vi "PickAndDestroy.vi"(0 "Image Settings":T3 {"2nd Axis" items=["x", "y", "z"]; "1st Axis" items=["x", "y", "z"]; "Time Resolution\n(ms/pixel)" format="%.2f"; "Image Resolution (nm/pixel)"."z" format="%.2f"; "Image Resolution (nm/pixel)"."y" format="%.2f"; "Image Resolution (nm/pixel)"."x" format="%.2f"; "Image Size (µm)"."z" format="%.2f"; "Image Size (µm)"."y" format="%.2f"; "Image Size (µm)"."x" format="%.2f"; "End Position (µm)"."z" format="%.2f"; "End Position (µm)"."y" format="%.2f"; "End Position (µm)"."x" format="%.2f"; "Start Position (µm)"."z" format="%.2f"; "Start Position (µm)"."y" format="%.2f"; "Start Position (µm)"."x" format="%.2f"}, 1 "Threshold":dbl=20.0 format="%.2f", 2 "Image":u32[][](array[numeric])) -> ()   [LabVIEW 2009]
uses:
  ImageSettings.ctt
  AO Update Channel.vi
  <vilib>/ptbypt/NI_PtbyPt.lvlib
panel:
  in  "AFM mode":bool
  in  "gauss fit":bool
  in  "channel":i32
  in  "initialize":bool
  out "Histogram Graph":T1(graph)
  in  ".sm file format":bool
  in  "manual positioning":cluster{"x":dbl, "y":dbl, "z":dbl}
  in  "Laser 4":bool
  out "used":bool
  in  "Ramp Setup":bool
  in  "% duration Laser1":u8=50 min=1 max=99
  in  "% puls-duration":dbl=100.0
  in  "Laser 3":bool
  in  "Laser 2":bool
  in  "Laser 1":bool
  in  "AOTF Setup":bool
  in  "AOTF":u16(ring)=1 items=["None", "Laser 1", "Laser 2", "Laser 1 + 2", "Laser 3", "Laser 1 + 3", "Laser 2 + 3", "Laser 1+2+3", "Laser 1+2+3+4", "Laser 2+3+4"]
  out "Pickcoord. (pixel)":cluster{dbl, dbl, dbl}
  in  "offset (pixel)":cluster{dbl, dbl, dbl}
  out "coordinates (pixel)":cluster{dbl, dbl, dbl}
  out "Actual Spot No.":u32
  in  "Store Pick Image":bool
  in  "Next":bool caption="Run"
  in  "Show MCS":bool=TRUE
  in  "Pick Settings":T2={"Automatic"=FALSE, "Threshold"=20.0, "radius"=0} {"Threshold" format="%.2f"}
  in  "Run":bool
  in  "Destination:":path
  in  "Store Data":bool caption="Store Data:"
  in  "Stage Setup":bool
  in  "SPC Setup":bool
  in  "EOM Setup":bool
  in  "EOM":u16(ring) items=["None", "Trace", "Retrace", "All"]
  out "Counts":cluster{"Total":u32, "Gap":u32, "Invalid":u32}
  out "MCS":i32[][](graph)
  in  "Exit":bool
  # "+"
  # "="
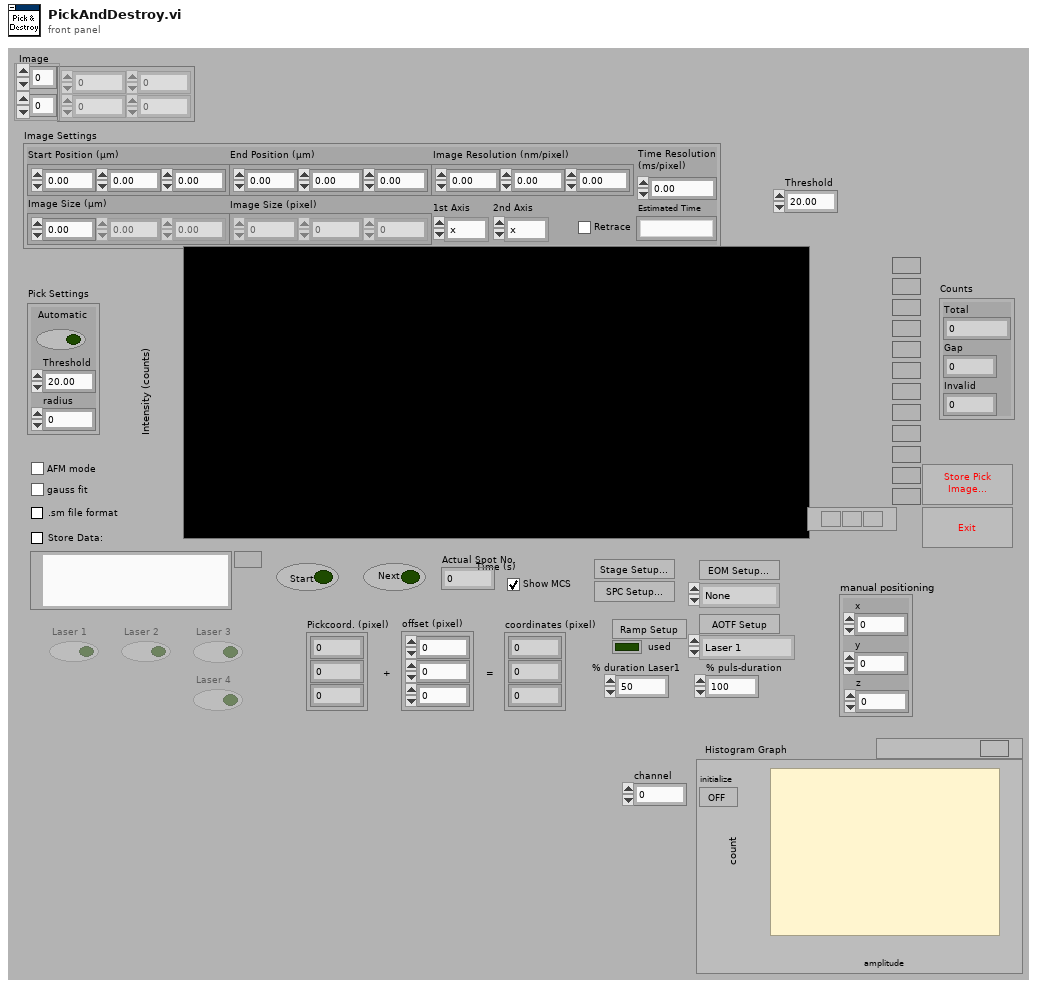
[diagram p1: front panel]
types:
  T1 = cluster{"X Values":dbl[], "Histogram: h(x)":i32[]}
  T2 = cluster{"Automatic":bool, "Threshold":dbl, "radius":i32}
  T3 = typedef "ImageSettings.ctt" = cluster{"Start Position (µm)":cluster{"x":dbl, "y":dbl, "z":dbl}, "End Position (µm)":cluster{"x":dbl, "y":dbl, "z":dbl}, "Image Resolution (nm/pixel)":cluster{"x":dbl, "y":dbl, "z":dbl}, "Image Size (µm)":cluster{"x":dbl, "y":dbl, "z":dbl}, "Image Size (pixel)":cluster{"x":u32, "y":u32, "z":u32}, "Time Resolution\n(ms/pixel)":dbl, "1st Axis":u16, "2nd Axis":u16, "Retrace":bool, "Estimated Time":string}
  T4 = enum16{"Get Type", "Set Type", "GetStageInit", "GetWriteStageSetting", "GetInitializeStageOutput", "GetSetAxisPosition", "GetSetPos", "GetSetupStage", "HaltStageOutput"}
  T5 = typedef "FIFOSettings.ctt" = cluster{"Measurement":cluster{"Binning (ms)":sgl, "External Trigger Condition":u16, "Stop Condition:":u16, "Stop Count":dbl, "Buffer Size (Photons)":u32, "No of Channels":u16, "Ext Latch Delay":i16}, "ADC":cluster{"Binning (HH)":i16, "Dither Range":i16, "Count Increment":i16, "Mode":u16}, "SYNC":cluster{"SYNC ZC Level (mV)":sgl, "SYNC Freq Divider":u16, "SYNC Holdoff (ps)":sgl, "SYNC Threshold (mV)":sgl}, "TAC":cluster{"TAC Range (ns)":sgl, "TAC Gain":i16, "TAC Offset (%)":sgl, "TAC Limit Low (%)":sgl, "TAC Limit High (%)":sgl}, "Ch 2":cluster{"Ch2 ZC Level (mV)":sgl, "Ch2 Holdoff (ps)":sgl, "Ch2 Threshold (mV)":sgl}, "Ch 3":cluster{"Ch3 ZC Level (mV)":sgl, "Ch3 Holdoff (ps)":sgl, "Ch3 Threshold (mV)":sgl}, "Ch 4":cluster{"Ch4 ZC Level (mV)":sgl, "Ch4 Holdoff (ps)":sgl, "Ch4 Threshold (mV)":sgl}, "Ch1":cluster{"Ch1 ZC Level (mV)":sgl, "Ch1 Holdoff (ps)":sgl, "Ch1 Threshold (mV)":sgl}}
  T6 = typedef "IMAQ Image.ctl" = refnum<image>
  T7 = typedef "PickImage.ctl" = cluster{"Rawdata":T6, "Mask":T6, "Display":T6, "Coefficients (2D)":sgl[][], "Destroy Index":u32}
  T8 = cluster{"Binning (ms)":sgl, "External Trigger Condition":u16, "Stop Condition:":u16, "Stop Count":dbl, "Buffer Size (Photons)":u32, "No of Channels":u16, "Ext Latch Delay":i16}
  T9 = cluster{"router channels":u8[], "macro times(50ns steps)":u32[], "micro times":u16[], "invalid times":u32[], "gap times":u32[]}
  T10 = cluster{"Start Position (µm)":cluster{"x":dbl, "y":dbl, "z":dbl}, "End Position (µm)":cluster{"x":dbl, "y":dbl, "z":dbl}, "Image Resolution (nm/pixel)":cluster{"x":dbl, "y":dbl, "z":dbl}, "Image Size (µm)":cluster{"x":dbl, "y":dbl, "z":dbl}, "Image Size (pixel)":cluster{"x":u32, "y":u32, "z":u32}, "Time Resolution\n(ms/pixel)":dbl, "1st Axis":u16, "2nd Axis":u16, "Retrace":bool, "Estimated Time":string}
  T11 = typedef "StageType.ctt" = enum16{"PI 725 USB", "PI 725 TCP/IP", "PI analogue step"}
  T12 = cluster{"used":bool, "steps":u16, "start (V)":dbl, "stop (V)":dbl, "periode (s)":dbl, "manual":dbl[][]}
  T13 = typedef "DAQLinescanVisualization.ctt" = cluster{"Threshold":u32, "Trace Window #":u32, "IMAQ Trace":T6, "Retrace Window #":u32, "IMAQ Retrace":T6}
  T14 = typedef "AOTFSettings.ctt" = cluster{"Laser 1 Output Channel":tag, "AOTF  1 Output Voltage":dbl, "Laser 2 Output Channel":tag, "AOTF  2 Output Voltage":dbl, "Laser 3 Output Channel":tag, "AOTF  3 Output Voltage":dbl, "Pixel per Cycle":u16, "Time per Cycle  / ms":dbl, "Laser 4 Output Channel":tag, "AOTF  4 Output Voltage":dbl, "Laser 5 Output Channel":tag, "AOTF 5 Output Voltage ":dbl, "Laser 6 Output Channel":tag, "AOTF  6 Output Voltage ":dbl, "Laser 7 Output Channel":tag, "AOTF 7 Output Voltage ":dbl, "Laser 8 Output Channel":tag, "AOTF  8 Output Voltage ":dbl, "AOTF  1 Frequency":dbl, "AOTF  2 Frequency":dbl, "AOTF  3  Frequency":dbl, "AOTF  4 Frequency":dbl, "AOTF 5 Frequency":dbl, "AOTF  6 Frequency":dbl, "AOTF 7  Frequency":dbl, "AOTF  8 Frequency":dbl, "AOTF  1 Amplitude":dbl, "AOTF  2 Amplitude":dbl, "AOTF  3  Amplitude":dbl, "AOTF  4 Amplitude":dbl, "AOTF 5 Amplitude":dbl, "AOTF  6 Amplitude":dbl, "AOTF 7 Amplitude  ":dbl, "AOTF  8 Amplitude":dbl}
  T15 = typedef "AnalogSettings.ctt" = cluster{"PCI 671x Device Number":u32, "Samples per Unit":u32}
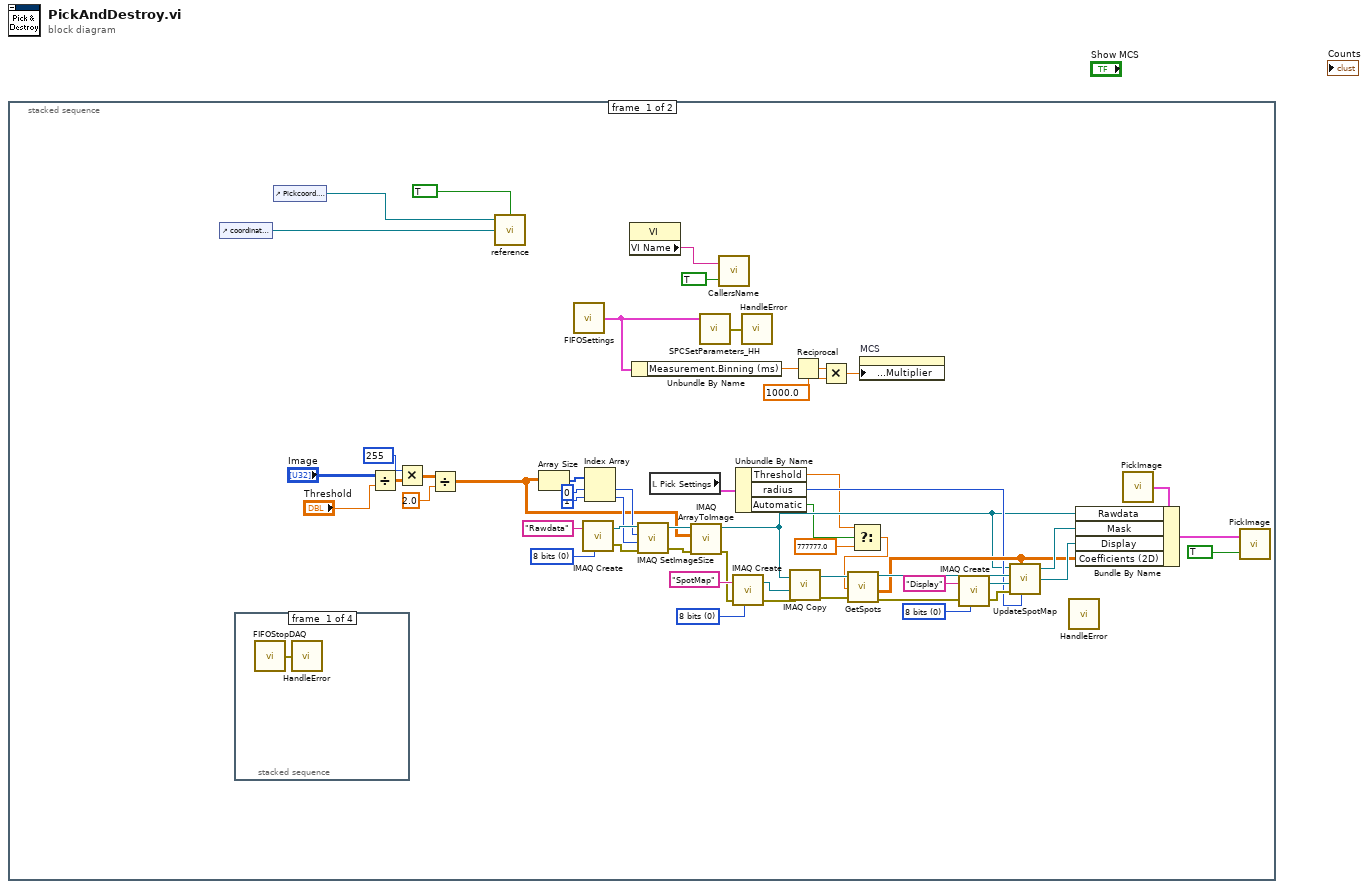
[diagram p0: block diagram]
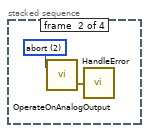
[diagram p2: hidden frame]
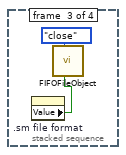
[diagram p3: hidden frame]
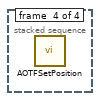
[diagram p4: hidden frame]
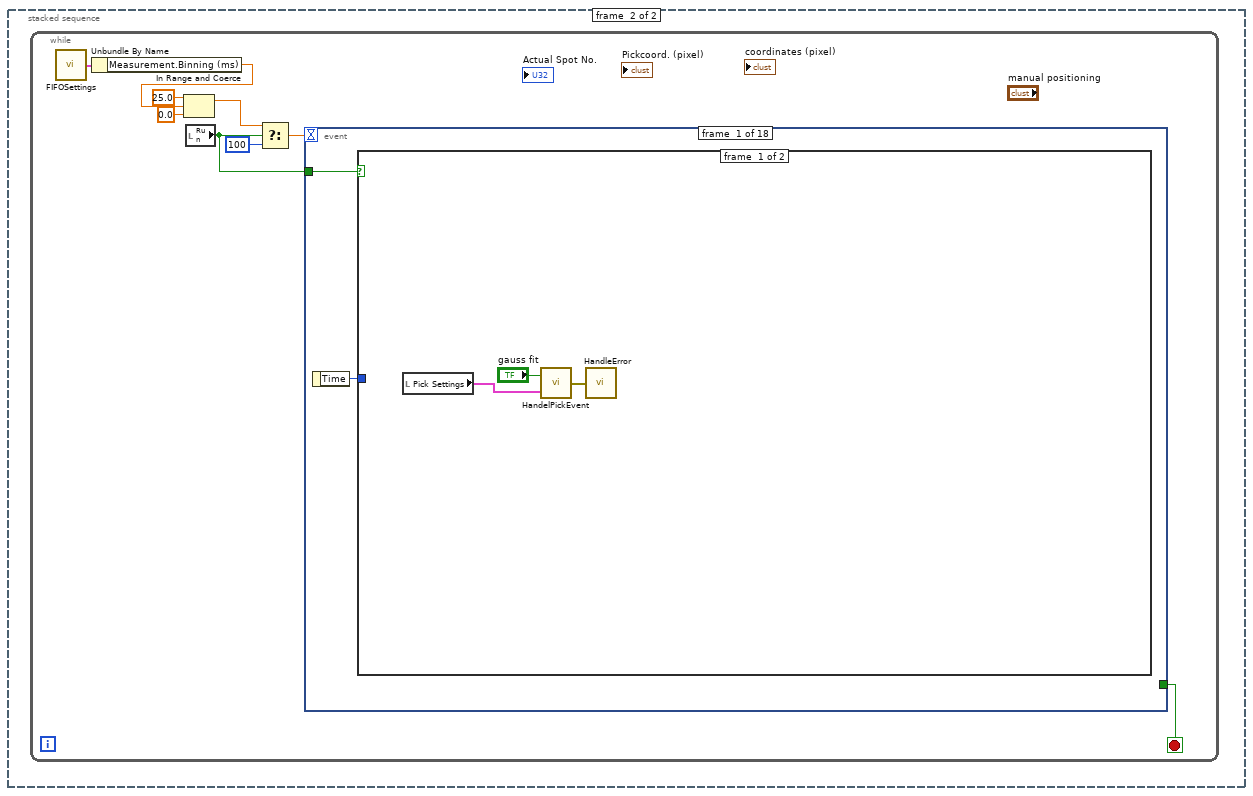
[diagram p5: hidden frame]
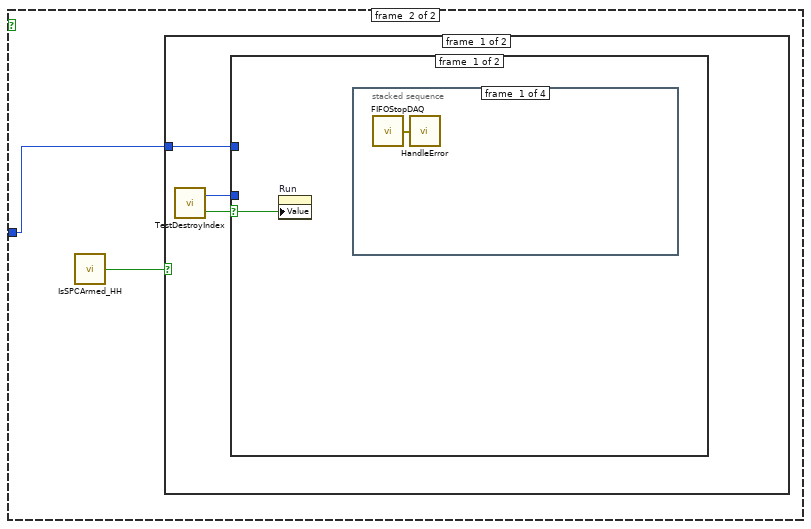
[diagram p6: hidden frame]
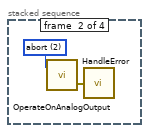
[diagram p7: hidden frame]
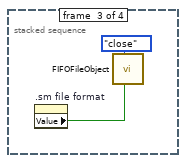
[diagram p8: hidden frame]
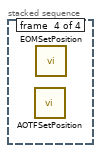
[diagram p9: hidden frame]
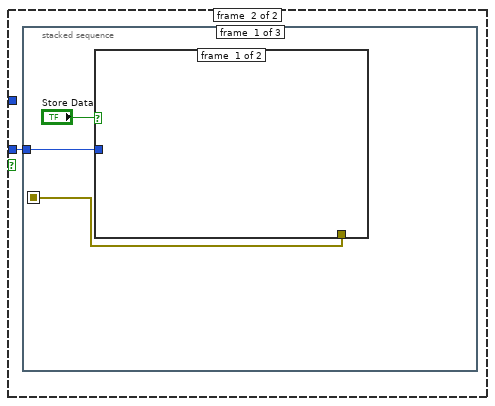
[diagram p10: hidden frame]
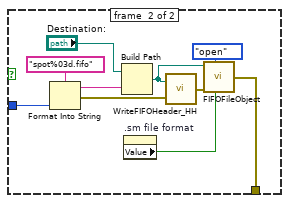
[diagram p11: hidden frame]
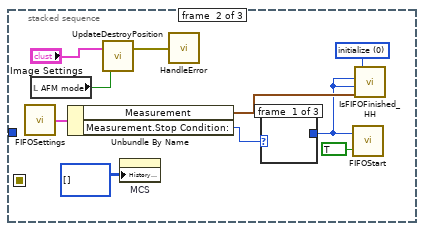
[diagram p12: hidden frame]
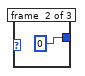
[diagram p13: hidden frame]
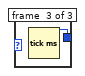
[diagram p14: hidden frame]
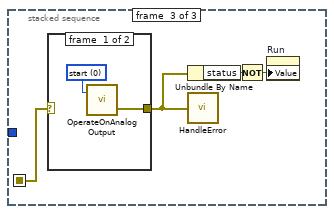
[diagram p15: hidden frame]
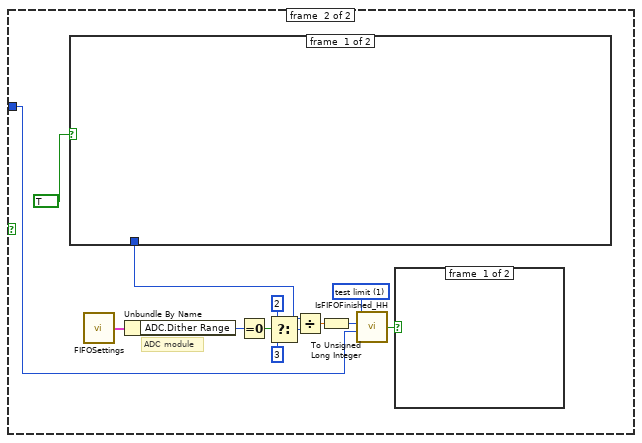
[diagram p17: hidden frame]
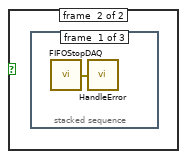
[diagram p18: hidden frame]
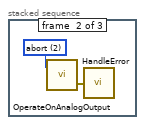
[diagram p19: hidden frame]
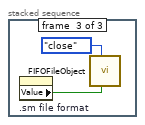
[diagram p20: hidden frame]
diagram:
  n1 = stacked-sequence {
    frame #0 {
      w39 = u32 0 items=["8 bits", "16 bits", "Float", "Complex", "RGB", "HSL"] ("Image Type")
      w44 = u32 0 items=["8 bits", "16 bits", "Float", "Complex", "RGB", "HSL"] ("Image Type")
      w54 = u32 0 items=["8 bits", "16 bits", "Float", "Complex", "RGB", "HSL"] ("Image Type")
      n2 = control-ref of="coordinates (pixel)"() -> (w16:refnum<vi>)
      n3 = stacked-sequence {
        frame #0 {
          n4 = call "FIFOStopDAQ.vi"() -> ("error out"=w56:errorcluster)
          n5 = call "HandleError.vi"("error in (no error)"=w56) -> ()
        }
        frame #1 {
          w58 = u16 2 items=["start", "state", "abort"] ("operation")
          n6 = call "OperateOnAnalogOutput.vi"("operation"=w58) -> ("error out"=w57:errorcluster)  [unwired: 1 in, 1 out]
          n7 = call "HandleError.vi"("error in (no error)"=w57) -> ()
        }
        frame #2 {
          n8 = property on=".sm file format" class="Bool (strict)"() -> ("Value"=w59:bool)  [unwired: 2 in, 2 out]
          n9 = call "FIFOFileObject.vi"(".sm file format"=w59, "function (open:0)"=enum16{"open", "write", "close"}."close") -> ()  [unwired: 4 in, 1 out]
        }
        frame #3 {
          n10 = call "AOTFSetPosition.vi"() -> ()  [unwired: 2 in]
        }
      }
      n11 = control-ref of="Pickcoord. (pixel)"() -> (w17:refnum<vi>)
      n12 = Divide(x="Image", y="Threshold") -> (x/y=w22:dbl[][])
      n13 = Multiply(x=u8 255, y=w22) -> (x*y=w7:dbl[][])
      n14 = Divide(x=w7, y=2.0) -> (x/y=w5:dbl[][])
      n15 = call "reference.vi"("set?"=TRUE, "coordinates (pixel)"=w16, "Pickcoord. (pixel)"=w17) -> ()  [unwired: 1 in, 2 out]
      n16 = Array Size(array=w5) -> (size(s)=w53:i32[])
      n17 = call "FIFOSettings.vi"() -> ("FIFO Settings(out)"=w14:T5)  [unwired: 2 in]
      n18 = call "IMAQ Create"("Image Name"="Rawdata", "Image Type"=w54) -> ("New Image"=w50:T6, "error out"=w49:errorcluster)  [unwired: 3 in]
      n19 = Index Array(array=w53, index #1=0 ("index"), index #2=1 ("index")) -> (element #1=w8:i32, element #2=w38:i32)
      n20 = property class="VI"() -> ("VI Name"=w18:string)  [unwired: 2 in, 2 out]
      n21 = Unbundle By Name(w14) -> ("Measurement.Binning (ms)"=w13:sgl)
      n22 = call "IMAQ SetImageSize"("error in (no error)"=w49, "Y Resolution"=w38, "X Resolution"=w8, "Image"=w50) -> ("error out"=w47:errorcluster, "Image Out"=w48:T6)  [unwired: 1 in]
      n23 = local read "Pick Settings"() -> (w26:T2)
      n24 = call "IMAQ ArrayToImage"("error in (no error)"=w47, "Image Pixels (U8)"=w5, "Image"=w48) -> ("error out"=w41:errorcluster, "Image Out"=w9:T6)  [unwired: 7 in]
      n25 = call "SPCSetParameters_HH.vi"("FIFO Settings"=w14) -> ("error (out)"=w24:errorcluster)  [unwired: 2 in]
      n26 = call "CallersName.vi"("Get/Set"=TRUE ("s"), "Callers Name"=w18) -> ()  [unwired: 1 out]
      n27 = call "IMAQ Create"("Image Name"="SpotMap", "Image Type"=w44, "error in (no error)"=w41) -> ("New Image"=w37:T6, "error out"=w36:errorcluster)  [unwired: 2 in]
      n28 = Unbundle By Name(w26) -> ("Threshold"=w4:dbl, "radius"=w25:i32, "Automatic"=w3:bool)
      n29 = call "HandleError.vi"("error in (no error)"=w24) -> ()
      n30 = call "IMAQ Copy"("error in (no error)"=w36, "Image Dst"=w37, "Image Src"=w9) -> ("error out"=w34:errorcluster, "Image Dst Out"=w35:T6)  [unwired: 3 in]
      n31 = Reciprocal(x=w13) -> (1/x=w12:sgl)
      n32 = Multiply(x=w12, y=sgl 1000.0) -> (x*y=w11:sgl)
      n33 = Select(t=w4, s=w3, f=777777.0) -> (s? t:f=w1:dbl)
      n34 = call "GetSpots.vi"("New Image"=w35, "Threshold"=w1, "error in (no error)"=w34) -> ("Image Dst Out"=w30:T6, "Coefficients (2D)"=w27:sgl[][], "error out"=w33:errorcluster)  [unwired: 2 out]
      n35 = property on="MCS" class="WFChart (strict)"("X Scale.Offset and Multiplier:Multiplier"=w11) -> ()  [unwired: 2 in, 2 out]
      n36 = call "IMAQ Create"("Image Name"="Display", "Image Type"=w39, "error in (no error)"=w33) -> ("New Image"=w31:T6, "error out"=w32:errorcluster)  [unwired: 2 in]
      n37 = call "UpdateSpotMap.vi"("Rawdata"=w9, "Coefficients"=w27, "Mask (input)"=w30, "Display Input"=w31, "radius"=w25, "error in (no error)"=w32) -> ("Mask (output)"=w29:T6, "Display (output"=w28:T6)  [unwired: 1 out]
      n38 = call "HandleError.vi"() -> ()  [unwired: 1 in]
      n39 = call "PickImage.vi"() -> ("Image (output)"=w46:T7)  [unwired: 2 in]
      n40 = Bundle By Name(cluster=w46, "Rawdata"=w9, "Mask"=w29, "Display"=w28, "Coefficients (2D)"=w27) -> (w42:T7)
      n41 = call "PickImage.vi"("Get/Set"=TRUE, "Images (input)"=w42) -> ()  [unwired: 1 out]
    }
    frame #1 {
      n42 = while {
        stop <- w69 stop-if-true
        n43 = call "FIFOSettings.vi"() -> ("FIFO Settings(out)"=w65:T5)  [unwired: 2 in]
        n44 = Unbundle By Name(w65) -> ("Measurement.Binning (ms)"=w62:sgl)
        n45 = In Range and Coerce(upper limit=25.0, x=w62, lower limit=0.0) -> (coerced(x)=w61:dbl)  [unwired: 1 out]
        n46 = local read "Run"() -> (w66:bool)
        n47 = Select(t=w61, s=w66, f=100) -> (s? t:f=w67:dbl)
        n48 = event shown="[10] \"Run\": Value Change" {
          selector: _ -> [_ _ _ _ _ _ _ _ _ _ _ _ _ _ _ _ _ _]
          dyn-events: _ -> [_ _ _ _ _ _ _ _ _ _ _ _ _ _ _ _ _ _]
          timeout: w67 -> [_ _ _ _ _ _ _ _ _ _ _ _ _ _ _ _ _ _]
          tunnel: [_ _ _ _ _ _ _ _ _ _ _ _ _ _ _ _ _ TRUE] -> w69
          tunnel: w66 -> [w71 _ _ _ _ _ _ _ _ _ _ _ _ _ _ _ _ _]
          event #0 {
            n49 = event-data() -> ("Time"=w70:u32)  [unwired: 1 in]
            n50 = case shown="True" w71 {
              tunnel: w70 -> [_ w75]
              frame #0 {
                n51 = local read "Pick Settings"() -> (w74:T2)
                n52 = call "HandelPickEvent.vi"("Pick Settings"=w74, "gauss fit"="gauss fit") -> ("error out"=w73:errorcluster)
                n53 = call "HandleError.vi"("error in (no error)"=w73) -> ()
              }
              frame #1 {
                n54 = call "IsSPCArmed_HH.vi"() -> ("Boolean"=w76:bool)  [unwired: 1 in]
                n55 = case shown="False" w76 {
                  tunnel: w75 -> [w79 w121]
                  frame #0 {
                    n56 = call "TestDestroyIndex.vi"() -> ("Boolean"=w78:bool, "Destroy Index"=w77:u32)
                    n57 = case shown="True" w78 {
                      selector: w78 -> [w80 _]
                      tunnel: w79 -> [_ _]
                      tunnel: w77 -> [_ w86]
                      frame #0 {
                        n58 = property on="Run" class="Boolean (strict)"("Value"=w80) -> ()  [unwired: 2 in, 2 out]
                        n59 = stacked-sequence {
                          frame #0 {
                            n60 = call "FIFOStopDAQ.vi"() -> ("error out"=w81:errorcluster)
                            n61 = call "HandleError.vi"("error in (no error)"=w81) -> ()
                          }
                          frame #1 {
                            w83 = u16 2 items=["start", "state", "abort"] ("operation")
                            n62 = call "OperateOnAnalogOutput.vi"("operation"=w83) -> ("error out"=w82:errorcluster)  [unwired: 1 in, 1 out]
                            n63 = call "HandleError.vi"("error in (no error)"=w82) -> ()
                          }
                          frame #2 {
                            n64 = property on=".sm file format" class="Bool (strict)"() -> ("Value"=w84:bool)  [unwired: 2 in, 2 out]
                            n65 = call "FIFOFileObject.vi"(".sm file format"=w84, "function (open:0)"=enum16{"open", "write", "close"}."close") -> ()  [unwired: 4 in, 1 out]
                          }
                          frame #3 {
                            n66 = call "AOTFSetPosition.vi"() -> ()  [unwired: 2 in]
                            n67 = call "EOMSetPosition.vi"() -> ()  [unwired: 1 in]
                          }
                        }
                      }
                      frame #1 {
                        n68 = stacked-sequence {
                          seq-local: [w88 _ _] -> [_ _ w115]
                          tunnel: w86 -> [w87 _ _]
                          frame #0 {
                            n69 = case shown="True" "Store Data" {
                              tunnel: [_ w97] -> w88
                              tunnel: w87 -> [_ w92]
                              frame #0 {
                              }
                              frame #1 {
                                n70 = Format Into String(format string="spot%03d.fifo", w92) -> (resulting string=w94:string, error out=w93:errorcluster)  [unwired: 2 in]
                                n71 = Build Path(base path="Destination:", name or relative path=w94) -> (appended path=w91:path)
                                n72 = property on=".sm file format" class="Bool (strict)"() -> ("Value"=w90:bool)  [unwired: 2 in, 2 out]
                                n73 = call "WriteFIFOHeader_HH.vi"("error in"=w93, "Destination:"=w91) -> ("error out"=w98:errorcluster)
                                n74 = call "FIFOFileObject.vi"(".sm file format"=w90, "function (open:0)"=enum16{"open", "write", "close"}."open", "error in (no error)"=w98, "Destination:"=w91) -> ("error out"=w97:errorcluster)  [unwired: 2 in]
                              }
                            }
                          }
                          frame #1 {
                            w105 = u16 0 items=["initialize", "test limit"] ("operation")
                            n75 = call "FIFOSettings.vi"() -> ("FIFO Settings(out)"=w106:T5)  [unwired: 2 in]
                            n76 = local read "AFM mode"() -> (w100:bool)
                            n77 = Unbundle By Name(w106) -> ("Measurement"=w104:T8, "Measurement.Stop Condition:"=w107:u16)
                            n78 = call "UpdateDestroyPosition.vi"("AFM Mode"=w100, "Image Settings"="Image Settings") -> ("error out"=w101:errorcluster)  [unwired: 1 in]
                            n79 = property on="MCS" class="WFChart (strict)"("History Data"=u32[][] []) -> ()  [unwired: 2 in, 2 out]
                            n80 = call "HandleError.vi"("error in (no error)"=w101) -> ()
                            n81 = case shown="2" w107 {
                              tunnel: [_ u32 0 ("Start (input)") w111] -> w102
                              frame #0 {
                              }
                              frame #1 {
                              }
                              frame #2 {
                                n82 = Tick Count (ms)() -> (millisecond timer value=w111:u32)
                              }
                            }
                            n83 = call "FIFOStart.vi"("Set/Get"=TRUE, "Start (input)"=w102) -> ()  [unwired: 1 out]
                            n84 = call "IsFIFOFinished_HH.vi"("Measurement"=w104, "Time"=w102, "Counts"=w102, "operation"=w105) -> ()  [unwired: 1 out]
                          }
                          frame #2 {
                            n85 = case shown="No Error" w115 {
                              selector: w115 -> [_ w118]
                              tunnel: [w116 w118] -> w112
                              frame #0 {
                                w117 = u16 0 items=["start", "state", "abort"] ("operation")
                                n86 = call "OperateOnAnalogOutput.vi"("operation"=w117) -> ("error out"=w116:errorcluster)  [unwired: 1 in, 1 out]
                              }
                              frame #1 {
                              }
                            }
                            n87 = Unbundle By Name(w112) -> ("status"=w114:bool)
                            n88 = call "HandleError.vi"("error in (no error)"=w112) -> ()
                            n89 = Not(x=w114) -> (.not. x?=w113:bool)
                            n90 = property on="Run" class="Boolean (strict)"("Value"=w113) -> ()  [unwired: 2 in, 2 out]
                          }
                        }
                      }
                    }
                  }
                  frame #1 {
                    w131 = u16 1 items=["initialize", "test limit"] ("operation")
                    # "ADC module"
                    n91 = case shown="True" TRUE ("Case Constant\n(See Context Help)") {
                      tunnel: [_ w144] -> w120
                      frame #0 {
                      }
                      frame #1 {
                        w143 = u16 1 items=["init", "run"] ("mode")
                        n92 = property on=".sm file format" class="Bool (strict)"() -> ("Value"=w149:bool)  [unwired: 2 in, 2 out]
                        n93 = property on="Store Data" class="Boolean (strict)"() -> ("Value"=w150:bool)  [unwired: 2 in, 2 out]
                        n94 = call "SPCReadFIFO_HH.vi"() -> ("count"=w144:i32, "error out"=w151:errorcluster, "buffer"=w145:u32[])  [unwired: 2 in]
                        n95 = case shown="False" w150 {
                          tunnel: [w160 w166] -> w152
                          tunnel: w151 -> [w160 w165]
                          tunnel: w145 -> [_ w163]
                          tunnel: w144 -> [_ w162]
                          tunnel: w149 -> [_ w161]
                          frame #0 {
                          }
                          frame #1 {
                            n96 = call "FIFOFileObject.vi"(".sm file format"=w161, "function (open:0)"=enum16{"open", "write", "close"}."write", "error in (no error)"=w165, "count"=w162, "buffer"=w163) -> ("error out"=w166:errorcluster)  [unwired: 1 in]
                          }
                        }
                        n97 = Array Subset(array=w145, index=0, length=w144) -> (w147:u32[])
                        n98 = call "ParseFIFO_HH.vi"("RawData"=w147) -> ("RawData Out"=w146:T9)  [unwired: 1 in]
                        n99 = call "HandleError.vi"("error in (no error)"=w152) -> ()
                        n100 = call "_updateOnlineDisplay_LV.vi"("show lifetime"=FALSE, "Raw Data"=w146, "mode"=w143) -> ("Timetraces"=w141:i32[][])  [unwired: 1 in, 1 out]
                        "MCS" <- w141
                        n101 = Index Array(array=w141, index (row)="channel") -> (element=w139:i32[])  [unwired: 1 in]
                        n102 = for {
                          tunnel: w139 -> [w155] mode=indexing
                          tunnel: 1000 ("sample length") -> [w158]
                          tunnel: "initialize" -> [w157]
                          n103 = call <vilib>:"Histogram PtByPt.vi"("initialize"=w157, "sample length"=w158, "intervals"=10, "x"=w155) -> ("Histogram Graph"=→"Histogram Graph":T1)  [unwired: 4 in, 3 out]
                          n104 = Equal To 0?(x=w155) -> (x = 0?=w154:bool)
                          n105 = case shown="False" w154 {
                            tunnel: w154 -> [_ w159]
                            tunnel: [_ w159] -> _
                            frame #0 {
                            }
                            frame #1 {
                            }
                          }
                        }
                      }
                    }
                    n106 = call "FIFOSettings.vi"() -> ("FIFO Settings(out)"=w129:T5)  [unwired: 2 in]
                    n107 = Unbundle By Name(w129) -> ("ADC.Dither Range"=w123:i16)
                    n108 = Equal To 0?(x=w123) -> (x = 0?=w124:bool)
                    n109 = Select(t=2, s=w124, f=3) -> (s? t:f=w127:i32)
                    n110 = Divide(x=w120, y=w127) -> (x/y=w128:dbl)
                    n111 = To Unsigned Long Integer(number=w128) -> (unsigned 32bit integer=w130:u32)
                    n112 = call "IsFIFOFinished_HH.vi"("Time"=w121, "Counts"=w130, "operation"=w131) -> ("Boolean"=w122:bool)  [unwired: 1 in]
                    n113 = case shown="False" w122 {
                      frame #0 {
                      }
                      frame #1 {
                        n114 = stacked-sequence {
                          frame #0 {
                            n115 = call "FIFOStopDAQ.vi"() -> ("error out"=w132:errorcluster)
                            n116 = call "HandleError.vi"("error in (no error)"=w132) -> ()
                          }
                          frame #1 {
                            w134 = u16 2 items=["start", "state", "abort"] ("operation")
                            n117 = call "OperateOnAnalogOutput.vi"("operation"=w134) -> ("error out"=w133:errorcluster)  [unwired: 1 in, 1 out]
                            n118 = call "HandleError.vi"("error in (no error)"=w133) -> ()
                          }
                          frame #2 {
                            n119 = property on=".sm file format" class="Bool (strict)"() -> ("Value"=w135:bool)  [unwired: 2 in, 2 out]
                            n120 = call "FIFOFileObject.vi"(".sm file format"=w135, "function (open:0)"=enum16{"open", "write", "close"}."close") -> ()  [unwired: 4 in, 1 out]
                          }
                        }
                      }
                    }
                  }
                }
              }
            }
          }
          event #1 {
            n121 = event-data() -> ()  [unwired: 1 in, 5 out]
            n122 = stacked-sequence {
              frame #0 {
                n123 = call "PickImage.vi"() -> ("Image (output)"=w170:T7)  [unwired: 2 in]
                n124 = Unbundle By Name(w170) -> ("Destroy Index"=w168:u32)
                n125 = stacked-sequence {
                  frame #0 {
                    n126 = call "FIFOStopDAQ.vi"() -> ("error out"=w172:errorcluster)
                    n127 = call "HandleError.vi"("error in (no error)"=w172) -> ()
                  }
                  frame #1 {
                    w174 = u16 2 items=["start", "state", "abort"] ("operation")
                    n128 = call "OperateOnAnalogOutput.vi"("operation"=w174) -> ("error out"=w173:errorcluster)  [unwired: 1 in, 1 out]
                    n129 = call "HandleError.vi"("error in (no error)"=w173) -> ()
                  }
                  frame #2 {
                    n130 = property on=".sm file format" class="Bool (strict)"() -> ("Value"=w175:bool)  [unwired: 2 in, 2 out]
                    n131 = call "FIFOFileObject.vi"(".sm file format"=w175, "function (open:0)"=enum16{"open", "write", "close"}."close") -> ()  [unwired: 4 in, 1 out]
                  }
                  frame #3 {
                    n132 = property on="EOM" class="Ring (strict)"() -> ("Value"=w179:u16)  [unwired: 2 in, 2 out]
                    n133 = property on="AOTF" class="Ring (strict)"() -> ("Value"=w177:u16)  [unwired: 2 in, 2 out]
                    n134 = Equal To 0?(x=w179) -> (x = 0?=w180:bool)
                    n135 = Equal To 0?(x=w177) -> (x = 0?=w178:bool)
                    n136 = case shown="True" w180 {
                      frame #0 {
                        n137 = call "EOMSetPosition.vi"("value"=sgl 0.0) -> ()
                      }
                      frame #1 {
                      }
                    }
                    n138 = case shown="False" w178 {
                      frame #0 {
                        n139 = call "AOTFSetPosition.vi"() -> ()  [unwired: 2 in]
                      }
                      frame #1 {
                      }
                    }
                  }
                }
                n140 = Increment(x=w168) -> (x+1=w169:u32)
                n141 = Bundle By Name(cluster=w170, "Destroy Index"=w169) -> (w171:T7)
                n142 = call "PickImage.vi"("Get/Set"=TRUE, "Images (input)"=w171) -> ()  [unwired: 1 out]
              }
              frame #1 {
                n143 = call "TestDestroyIndex.vi"() -> ("Boolean"=w183:bool, "Destroy Index"=w182:u32)
                n144 = case shown="True" w183 {
                  tunnel: w182 -> [_ w186]
                  frame #0 {
                    w184 = FALSE ("Laser 1")
                    n145 = call "AOTFSetPosition.vi"() -> ()  [unwired: 2 in]
                    n146 = property on="Run" class="Bool (strict)"("Value"=FALSE ("Run")) -> ()  [unwired: 2 in, 2 out]
                    n147 = property on="Laser 1" class="Boolean (strict)"("Value"=w184) -> ()  [unwired: 2 in, 2 out]
                    n148 = property on="Laser 2" class="Boolean (strict)"("Value"=w184) -> ()  [unwired: 2 in, 2 out]
                    n149 = property on="Laser 3" class="Boolean (strict)"("Value"=w184) -> ()  [unwired: 2 in, 2 out]
                    n150 = property on="Laser 4" class="Boolesch (strikt)"("Value"=w184) -> ()  [unwired: 2 in, 2 out]
                  }
                  frame #1 {
                    n151 = stacked-sequence {
                      seq-local: [_ w190 _ _] -> [_ _ _ w218]
                      tunnel: w186 -> [w187 w188 _ _]
                      frame #0 {
                        n152 = property on="Actual Spot No." class="Digital (strict)"("Value"=w187) -> ()  [unwired: 2 in, 2 out]
                      }
                      frame #1 {
                        n153 = property on="Store Data" class="Boolean (strict)"() -> ("Value"=w189:bool)  [unwired: 2 in, 2 out]
                        n154 = case shown="False" w189 {
                          tunnel: [_ w198] -> w190
                          tunnel: w188 -> [_ w193]
                          frame #0 {
                          }
                          frame #1 {
                            n155 = property on="Destination:" class="Path"() -> ("Value"=w194:path)  [unwired: 2 in, 2 out]
                            n156 = Format Into String(format string="spot%03d.fifo", w193) -> (resulting string=w196:string, error out=w195:errorcluster)  [unwired: 2 in]
                            n157 = Build Path(base path=w194, name or relative path=w196) -> (appended path=w192:path)
                            n158 = property on=".sm file format" class="Bool (strict)"() -> ("Value"=w191:bool)  [unwired: 2 in, 2 out]
                            n159 = call "WriteFIFOHeader_HH.vi"("error in"=w195, "Destination:"=w192) -> ("error out"=w199:errorcluster)
                            n160 = call "FIFOFileObject.vi"(".sm file format"=w191, "function (open:0)"=enum16{"open", "write", "close"}."open", "error in (no error)"=w199, "Destination:"=w192) -> ("error out"=w198:errorcluster)  [unwired: 2 in]
                          }
                        }
                      }
                      frame #2 {
                        w207 = u16 0 items=["initialize", "test limit"] ("operation")
                        n161 = property on="Image Settings" class="Cluster (strict)"() -> ("Value"=w203:T10)  [unwired: 2 in, 2 out]
                        n162 = local read "AFM mode"() -> (w201:bool)
                        n163 = call "FIFOSettings.vi"() -> ("FIFO Settings(out)"=w208:T5)  [unwired: 2 in]
                        n164 = Unbundle By Name(w208) -> ("Measurement"=w206:T8, "Measurement.Stop Condition:"=w209:u16)
                        n165 = call "UpdateDestroyPosition.vi"("AFM Mode"=w201, "Image Settings"=w203) -> ("error out"=w202:errorcluster)  [unwired: 1 in]
                        n166 = property on="MCS" class="WFChart (strict)"("History Data"=u32[][] []) -> ()  [unwired: 2 in, 2 out]
                        n167 = call "HandleError.vi"("error in (no error)"=w202) -> ()
                        n168 = case shown="2" w209 {
                          tunnel: [_ u32 0 ("Start (input)") w212] -> w204
                          frame #0 {
                          }
                          frame #1 {
                          }
                          frame #2 {
                            n169 = Tick Count (ms)() -> (millisecond timer value=w212:u32)
                          }
                        }
                        n170 = call "FIFOStart.vi"("Set/Get"=TRUE, "Start (input)"=w204) -> ()  [unwired: 1 out]
                        n171 = call "IsFIFOFinished_HH.vi"("Measurement"=w206, "Time"=w204, "Counts"=w204, "operation"=w207) -> ()  [unwired: 1 out]
                      }
                      frame #3 {
                        n172 = call "StageType.vi"("Function"=T4."Get Type") -> ("Stage Type (output)"=w213:T11)  [unwired: 2 in, 2 out]
                        n173 = case shown="No Error" w218 {
                          selector: w218 -> [_ w224]
                          tunnel: [w220 w224] -> w215
                          tunnel: w213 -> [w219 _]
                          frame #0 {
                            n174 = case shown="\"PI 725 TCP/IP\", Default" w219 {
                              tunnel: [w221 w222] -> w220
                              frame #0 {
                                n175 = call "FIFOStartDAQ_HH.vi"() -> ("error out"=w221:errorcluster)  [unwired: 1 in]
                              }
                              frame #1 {
                                w223 = u16 0 items=["start", "state", "abort"] ("operation")
                                n176 = call "OperateOnAnalogOutput.vi"("operation"=w223) -> ("error out"=w222:errorcluster)  [unwired: 1 in, 1 out]
                              }
                            }
                          }
                          frame #1 {
                          }
                        }
                        n177 = Unbundle By Name(w215) -> ("status"=w217:bool)
                        n178 = call "HandleError.vi"("error in (no error)"=w215) -> ()
                        n179 = Not(x=w217) -> (.not. x?=w216:bool)
                        n180 = property on="Run" class="Bool (strict)"("Value"=w216) -> ()  [unwired: 2 in, 2 out]
                      }
                    }
                  }
                }
              }
            }
          }
          event #2 {
            n181 = event-data() -> ()  [unwired: 1 in, 5 out]
            n182 = call "PickImage.vi"() -> ("Image (output)"=w226:T7)  [unwired: 2 in]
            n183 = stacked-sequence {
              tunnel: w226 -> [_ w247 _]
              tunnel: "Pick Settings" -> [w228 _ w248]
              frame #0 {
                n184 = Bundle By Name(cluster=w228, "Automatic"=TRUE) -> (w229:T2)
                n185 = local write "Pick Settings"(w229) -> ()
              }
              frame #1 {
                n186 = local read "Pick Settings"() -> (w232:T2)
                n187 = Unbundle By Name(w247) -> ("Rawdata"=w240:T6, "Mask"=w241:T6, "Display"=w238:T6)
                n188 = Unbundle By Name(w232) -> ("Threshold"=w231:dbl, "radius"=w230:i32)
                n189 = call "IMAQ Copy"("Image Dst"=w241, "Image Src"=w240) -> ("error out"=w242:errorcluster, "Image Dst Out"=w243:T6)  [unwired: 4 in]
                n190 = call "GetSpots.vi"("New Image"=w243, "Threshold"=w231, "error in (no error)"=w242) -> ("Image Dst Out"=w239:T6, "Coefficients (2D)"=w233:sgl[][], "error out"=w237:errorcluster)  [unwired: 2 out]
                n191 = call "UpdateSpotMap.vi"("Rawdata"=w240, "Coefficients"=w233, "Mask (input)"=w239, "Display Input"=w238, "radius"=w230, "error in (no error)"=w237) -> ("Mask (output)"=w236:T6, "Display (output"=w235:T6, "error out"=w234:errorcluster)
                n192 = call "HandleError.vi"("error in (no error)"=w234) -> ()
                n193 = call "PickImage.vi"() -> ("Image (output)"=w246:T7)  [unwired: 2 in]
                n194 = Bundle By Name(cluster=w246, "Mask"=w236, "Display"=w235, "Coefficients (2D)"=w233) -> (w244:T7)
                n195 = call "PickImage.vi"("Get/Set"=TRUE, "Images (input)"=w244) -> ()  [unwired: 1 out]
              }
              frame #2 {
                n196 = Bundle By Name(cluster=w248, "Automatic"=FALSE) -> (w250:T2)
                n197 = local write "Pick Settings"(w250) -> ()
              }
            }
          }
          event #3 {
            n198 = event-data() -> ()  [unwired: 1 in, 5 out]
            n199 = call "PickImage.vi"() -> ("Image (output)"=w263:T7)  [unwired: 2 in]
            n200 = Unbundle By Name(w263) -> ("Rawdata"=w258:T6, "Mask"=w257:T6, "Display"=w256:T6, "Coefficients (2D)"=w259:sgl[][])
            n201 = local read "Pick Settings"() -> (w252:T2)
            n202 = Unbundle By Name(w252) -> ("radius"=w251:i32)
            n203 = call "UpdateSpotMap.vi"("Rawdata"=w258, "Coefficients"=w259, "Mask (input)"=w257, "Display Input"=w256, "radius"=w251) -> ("Mask (output)"=w255:T6, "Display (output"=w254:T6, "error out"=w253:errorcluster)  [unwired: 1 in]
            n204 = call "HandleError.vi"("error in (no error)"=w253) -> ()
            n205 = call "PickImage.vi"() -> ("Image (output)"=w262:T7)  [unwired: 2 in]
            n206 = Bundle By Name(cluster=w262, "Mask"=w255, "Display"=w254) -> (w260:T7)
            n207 = call "PickImage.vi"("Get/Set"=TRUE, "Images (input)"=w260) -> ()  [unwired: 1 out]
          }
          event #4 {
            n208 = event-data() -> ()  [unwired: 1 in, 5 out]
            n209 = stacked-sequence {
              frame #0 {
                w264 = u16 1 items=["standalone", "dialog"] ("mode")
                n210 = call "DAQFIFO_HH.vi"("mode"=w264) -> ()
              }
              frame #1 {
                n211 = call "FIFOSettings.vi"() -> ("FIFO Settings(out)"=w265:T5)  [unwired: 2 in]
                n212 = Unbundle By Name(w265) -> ("Measurement.Binning (ms)"=w269:sgl)
                n213 = call "SPCSetParameters_HH.vi"("FIFO Settings"=w265) -> ("error (out)"=w270:errorcluster)  [unwired: 2 in]
                n214 = call "HandleError.vi"("error in (no error)"=w270) -> ()
                n215 = Reciprocal(x=w269) -> (1/x=w268:sgl)
                n216 = Multiply(x=w268, y=sgl 1000.0) -> (x*y=w267:sgl)
                n217 = property on="MCS" class="WFChart (strict)"("X Scale.Offset and Multiplier:Multiplier"=w267) -> ()  [unwired: 2 in, 2 out]
              }
            }
          }
          event #5 {
            n218 = event-data() -> ()  [unwired: 1 in, 5 out]
            n219 = call "SetupEOM.vi"() -> ()  [unwired: 1 in]
          }
          event #6 {
            n220 = event-data() -> ()  [unwired: 1 in, 6 out]
            n221 = call "SetupAOTF.vi"() -> ()  [unwired: 1 in]
          }
          event #7 {
            n222 = event-data() -> ()  [unwired: 1 in, 5 out]
            n223 = case shown="True" "Stage Setup" {
              frame #0 {
              }
              frame #1 {
                n224 = stacked-sequence {
                  seq-local: [w272 _ _] -> [_ _ w274]
                  frame #0 {
                    n225 = call "StageType.vi"() -> ("Stage Type (output)"=w272:T11)  [unwired: 3 in, 2 out]
                  }
                  frame #1 {
                    n226 = call "SetupStage.vi"() -> ()  [unwired: 1 in]
                  }
                  frame #2 {
                    n227 = call "StageType.vi"() -> ("Stage Type (output)"=w275:T11)  [unwired: 3 in, 2 out]
                    n228 = Not Equal?(x=w274, y=w275) -> (x != y?=w273:bool)
                    n229 = case shown="True" w273 {
                      frame #0 {
                      }
                      frame #1 {
                        n230 = call "StageInit.vi"() -> ("error out"=w276:errorcluster)  [unwired: 1 in]
                        n231 = call "HandleError.vi"("error in (no error)"=w276) -> ()
                      }
                    }
                  }
                }
              }
            }
          }
          event #8 {
            n232 = event-data() -> ()  [unwired: 1 in, 6 out]
            n233 = flat-sequence {
              frame #0 {
                n234 = call "RampSetup.vi"() -> ()  [unwired: 1 in]
              }
              frame #1 {
                n235 = call "RampSetting.vi"() -> ("RampSetting (out)"=w278:T12)  [unwired: 2 in]
                n236 = Unbundle By Name(w278) -> ("used"=→"used":bool)
              }
            }
          }
          event #9 {
            n237 = event-data() -> ()  [unwired: 1 in, 5 out]
            n238 = call "PickImage.vi"() -> ("Image (output)"=w280:T7)  [unwired: 2 in]
            n239 = Unbundle By Name(w280) -> ("Display"=w279:T6)
            n240 = call "SaveIMAQImage.vi"("IMAQ Image"=w279) -> ()
          }
          event #10 {
            n241 = event-data() -> ()  [unwired: 1 in, 5 out]
            n242 = case shown="True" "Run" {
              frame #0 {
                w283 = FALSE ("Laser 1")
                n243 = property on=".sm file format" class="Bool (strict)"() -> ("Value"=w282:bool)  [unwired: 2 in, 2 out]
                n244 = call "FIFOStopDAQ.vi"() -> ("error out"=w286:errorcluster)
                n245 = call "OperateOnAnalogOutput.vi"("error in (no error)"=w286, "operation"=enum16{"start", "state", "abort"}."abort") -> ("error out"=w285:errorcluster)  [unwired: 1 out]
                n246 = call "FIFOFileObject.vi"(".sm file format"=w282, "function (open:0)"=enum16{"open", "write", "close"}."close", "error in (no error)"=w285) -> ("error out"=w287:errorcluster)  [unwired: 3 in]
                n247 = call "AOTFSetPosition.vi"() -> ()  [unwired: 2 in]
                n248 = call "HandleError.vi"("error in (no error)"=w287) -> ()
                n249 = property on="Laser 2" class="Boolean (strict)"("Value"=w283) -> ()  [unwired: 2 in, 2 out]
                n250 = property on="Laser 3" class="Boolean (strict)"("Value"=w283) -> ()  [unwired: 2 in, 2 out]
                n251 = property on="Laser 1" class="Boolean (strict)"("Value"=w283) -> ()  [unwired: 2 in, 2 out]
                n252 = property on="Laser 4" class="Boolesch (strikt)"("Value"=w283) -> ()  [unwired: 2 in, 2 out]
              }
              frame #1 {
                n253 = stacked-sequence {
                  frame #0 {
                    n254 = flat-sequence {
                      frame #0 {
                        n255 = call "RampSetting.vi"() -> ("RampSetting (out)"=w290:T12)  [unwired: 2 in]
                        n256 = Unbundle By Name(w290) -> ("used"=w289:bool)
                        n257 = case shown="False" w289 {
                          tunnel: "AOTF" -> [w292 w296]
                          frame #0 {
                            n258 = call "InitializeAnalogOutputforPAD.vi"("AOTF"=w292, "% puls-duration"="% puls-duration", "% rel. duration"="% duration Laser1", "EOM"="EOM") -> ()
                          }
                          frame #1 {
                            n259 = call "InitializeAnalogOutputforPADwithRamp.vi"("AOTF"=w296) -> ()  [unwired: 3 in]
                          }
                        }
                      }
                      frame #1 {
                        w298 = u16 0 items=["init", "run"] ("mode")
                        w299 = u32 0 ("Destroy Index")
                        n260 = property on="Actual Spot No." class="Digital (strict)"("Value"=w299) -> ()  [unwired: 2 in, 2 out]
                        n261 = call "FIFOInitDAQ_HH.vi"() -> ()  [unwired: 1 in]
                        n262 = call "PickImage.vi"() -> ("Image (output)"=w302:T7)  [unwired: 2 in]
                        n263 = Bundle By Name(cluster=w302, "Destroy Index"=w299) -> (w301:T7)
                        n264 = call "PickImage.vi"("Get/Set"=TRUE, "Images (input)"=w301) -> ()  [unwired: 1 out]
                        n265 = call "_updateOnlineDisplay_LV.vi"("show lifetime"=FALSE, "mode"=w298) -> ()  [unwired: 2 in, 2 out]
                      }
                    }
                  }
                  frame #1 {
                    n266 = call "TestDestroyIndex.vi"() -> ("Boolean"=w303:bool, "Destroy Index"=w304:u32)
                    n267 = case shown="True" w303 {
                      tunnel: w304 -> [_ w306]
                      frame #0 {
                        n268 = property on="Run" class="Boolean (strict)"("Value"=FALSE ("Run")) -> ()  [unwired: 2 in, 2 out]
                      }
                      frame #1 {
                        n269 = stacked-sequence {
                          seq-local: [_ w310 _ _] -> [_ _ _ w338]
                          tunnel: w306 -> [w307 w308 _ _]
                          frame #0 {
                            n270 = property on="Actual Spot No." class="DigNum (strict)"("Value"=w307) -> ()  [unwired: 2 in, 2 out]
                          }
                          frame #1 {
                            n271 = property on="Store Data" class="Bool (strict)"() -> ("Value"=w309:bool)  [unwired: 2 in, 2 out]
                            n272 = case shown="True" w309 {
                              tunnel: [_ w318] -> w310
                              tunnel: w308 -> [_ w313]
                              frame #0 {
                              }
                              frame #1 {
                                n273 = property on="Destination:" class="Path"() -> ("Value"=w314:path)  [unwired: 2 in, 2 out]
                                n274 = Format Into String(format string="spot%03d.fifo", w313) -> (resulting string=w316:string, error out=w315:errorcluster)  [unwired: 2 in]
                                n275 = Build Path(base path=w314, name or relative path=w316) -> (appended path=w312:path)
                                n276 = call "WriteFIFOHeader_HH.vi"("error in"=w315, "Destination:"=w312) -> ("error out"=w319:errorcluster)
                                n277 = call "FIFOFileObject.vi"(".sm file format"=".sm file format", "function (open:0)"=enum16{"open", "write", "close"}."open", "error in (no error)"=w319, "Destination:"=w312) -> ("error out"=w318:errorcluster)  [unwired: 2 in]
                              }
                            }
                          }
                          frame #2 {
                            w327 = u16 0 items=["initialize", "test limit"] ("operation")
                            n278 = property on="Image Settings" class="Clust (strict)"() -> ("Value"=w323:T10)  [unwired: 2 in, 2 out]
                            n279 = call "FIFOSettings.vi"() -> ("FIFO Settings(out)"=w328:T5)  [unwired: 2 in]
                            n280 = Unbundle By Name(w328) -> ("Measurement"=w326:T8, "Measurement.Stop Condition:"=w329:u16)
                            n281 = call "UpdateDestroyPosition.vi"("AFM Mode"="AFM mode", "Image Settings"=w323) -> ("error out"=w322:errorcluster)  [unwired: 1 in]
                            n282 = property on="MCS" class="WFChart (strict)"("History Data"=u32[][] []) -> ()  [unwired: 2 in, 2 out]
                            n283 = call "HandleError.vi"("error in (no error)"=w322) -> ()
                            n284 = case shown="2" w329 {
                              tunnel: [_ u32 0 ("Start (input)") w332] -> w324
                              frame #0 {
                              }
                              frame #1 {
                              }
                              frame #2 {
                                n285 = Tick Count (ms)() -> (millisecond timer value=w332:u32)
                              }
                            }
                            n286 = call "FIFOStart.vi"("Set/Get"=TRUE, "Start (input)"=w324) -> ()  [unwired: 1 out]
                            n287 = call "IsFIFOFinished_HH.vi"("Measurement"=w326, "Time"=w324, "Counts"=w324, "operation"=w327) -> ()  [unwired: 1 out]
                          }
                          frame #3 {
                            n288 = call "StageType.vi"("Function"=T4."Get Type") -> ("Stage Type (output)"=w333:T11)  [unwired: 2 in, 2 out]
                            n289 = case shown="No Error" w338 {
                              selector: w338 -> [_ w344]
                              tunnel: [w340 w344] -> w335
                              tunnel: w333 -> [w339 _]
                              frame #0 {
                                n290 = case shown="\"PI 725 USB\", \"PI 725 TCP/IP\"" w339 {
                                tunnel: [w341 w343] -> w340
                                frame #0 {
                                w342 = u16 0 items=["start", "state", "abort"] ("operation")
                                n291 = call "OperateOnAnalogOutput.vi"("operation"=w342) -> ("error out"=w341:errorcluster)  [unwired: 1 in, 1 out]
                                }
                                frame #1 {
                                n292 = call "FIFOStartDAQ_HH.vi"() -> ("error out"=w343:errorcluster)  [unwired: 1 in]
                                }
                                }
                              }
                              frame #1 {
                              }
                            }
                            n293 = Unbundle By Name(w335) -> ("status"=w337:bool)
                            n294 = call "HandleError.vi"("error in (no error)"=w335) -> ()
                            n295 = Not(x=w337) -> (.not. x?=w336:bool)
                            n296 = property on="Run" class="Bool (strict)"("Value"=w336) -> ()  [unwired: 2 in, 2 out]
                          }
                        }
                      }
                    }
                  }
                  frame #2 {
                    n297 = property on="Store Data" class="Boolesch (strikt)"() -> ("Value"=w345:bool)  [unwired: 2 in, 2 out]
                    n298 = case shown="False" w345 {
                      frame #0 {
                      }
                      frame #1 {
                        n299 = call "DAQLinescanVisualization.vi"() -> ("Visualization (output)"=w351:T13)  [unwired: 2 in]
                        n300 = property on="Destination:" class="Pfad"() -> ("Value"=w348:path)  [unwired: 2 in, 2 out]
                        n301 = Unbundle By Name(w351) -> ("IMAQ Trace"=w350:T6)
                        n302 = Build Path(base path=w348, name or relative path="SpotMap.png" ("Name oder relativer Pfad")) -> (appended path=w349:path)
                        n303 = call "IMAQ WriteFile"("File Type"="png", "File Path"=w349, "Image"=w350) -> ()  [unwired: 5 in, 1 out]
                      }
                    }
                  }
                }
              }
            }
          }
          event #11 {
            n304 = event-data() -> ("NewVal"=w353:u16)  [unwired: 1 in, 5 out]
            n305 = Not Equal To 0?(x=w353) -> (x != 0?=w352:bool)
            n306 = case shown="True" w352 {
              frame #0 {
                w354 = u8 0 ("Disabled")
                n307 = property on="Laser 1" class="Boolean (strict)"("Disabled"=w354) -> ()  [unwired: 2 in, 2 out]
                n308 = property on="Laser 2" class="Bool (strict)"("Disabled"=w354) -> ()  [unwired: 2 in, 2 out]
                n309 = property on="Laser 3" class="Bool (strict)"("Disabled"=w354) -> ()  [unwired: 2 in, 2 out]
                n310 = property on="Laser 4" class="Boolesch (strikt)"("Disabled"=w354) -> ()  [unwired: 2 in, 2 out]
              }
              frame #1 {
                w356 = FALSE ("Laser 1")
                w355 = u8 2 ("Disabled")
                n311 = call "AOTFSetPosition.vi"() -> ()  [unwired: 2 in]
                n312 = property on="Laser 1" class="Boolean (strict)"("Disabled"=w355, "Value"=w356) -> ()  [unwired: 2 in, 2 out]
                n313 = property on="Laser 2" class="Boolean (strict)"("Disabled"=w355, "Value"=w356) -> ()  [unwired: 2 in, 2 out]
                n314 = property on="Laser 3" class="Boolean (strict)"("Disabled"=w355, "Value"=w356) -> ()  [unwired: 2 in, 2 out]
                n315 = property on="Laser 4" class="Boolesch (strikt)"("Disabled"=w355, "Value"=w356) -> ()  [unwired: 2 in, 2 out]
              }
            }
          }
          event #12 {
            n316 = event-data() -> ()  [unwired: 1 in, 6 out]
            n317 = call "AOTFSettings.vi"() -> ("AOTF Setting (Output)"=w361:T14)  [unwired: 2 in]
            n318 = call "AnalogSettings.vi"() -> ("Analog Settings (output)"=w362:T15)  [unwired: 2 in]
            n319 = Unbundle By Name(w362) -> ("PCI 671x Device Number"=w360:u32)
            n320 = Unbundle By Name(w361) -> ("Laser 1 Output Channel"=w359:tag, "AOTF  1 Output Voltage"=w358:dbl)
            n321 = case shown="False" "Laser 1" {
              tunnel: w360 -> [w363 w368]
              tunnel: w359 -> [w364 w367]
              tunnel: w358 -> [_ w366]
              frame #0 {
                n322 = call-poly "AO Update Channel (scaled value).vi"("value"=sgl 0.0, "channel (0)"=w364, "device"=w363) -> ()
              }
              frame #1 {
                n323 = call-poly "AO Update Channel (scaled value).vi"("value"=w366, "channel (0)"=w367, "device"=w368) -> ()
              }
            }
          }
          event #13 {
            n324 = event-data() -> ()  [unwired: 1 in, 6 out]
            n325 = call "AOTFSettings.vi"() -> ("AOTF Setting (Output)"=w373:T14)  [unwired: 2 in]
            n326 = call "AnalogSettings.vi"() -> ("Analog Settings (output)"=w374:T15)  [unwired: 2 in]
            n327 = Unbundle By Name(w374) -> ("PCI 671x Device Number"=w372:u32)
            n328 = Unbundle By Name(w373) -> ("Laser 2 Output Channel"=w371:tag, "AOTF  2 Output Voltage"=w370:dbl)
            n329 = case shown="False" "Laser 2" {
              tunnel: w372 -> [w375 w380]
              tunnel: w371 -> [w376 w379]
              tunnel: w370 -> [_ w378]
              frame #0 {
                n330 = call-poly "AO Update Channel (scaled value).vi"("value"=sgl 0.0, "channel (0)"=w376, "device"=w375) -> ()
              }
              frame #1 {
                n331 = call-poly "AO Update Channel (scaled value).vi"("value"=w378, "channel (0)"=w379, "device"=w380) -> ()
              }
            }
          }
          event #14 {
            n332 = event-data() -> ()  [unwired: 1 in, 6 out]
            n333 = call "AOTFSettings.vi"() -> ("AOTF Setting (Output)"=w384:T14)  [unwired: 2 in]
            n334 = call "AnalogSettings.vi"() -> ("Analog Settings (output)"=w385:T15)  [unwired: 2 in]
            n335 = Unbundle By Name(w385) -> ("PCI 671x Device Number"=w383:u32)
            n336 = Unbundle By Name(w384) -> ("Laser 3 Output Channel"=w382:tag, "AOTF  3 Output Voltage"=w381:dbl)
            n337 = case shown="False" "Laser 3" {
              tunnel: w383 -> [w387 w392]
              tunnel: w382 -> [w388 w391]
              tunnel: w381 -> [_ w390]
              frame #0 {
                n338 = call-poly "AO Update Channel (scaled value).vi"("value"=sgl 0.0, "channel (0)"=w388, "device"=w387) -> ()
              }
              frame #1 {
                n339 = call-poly "AO Update Channel (scaled value).vi"("value"=w390, "channel (0)"=w391, "device"=w392) -> ()
              }
            }
          }
          event #15 {
            n340 = event-data() -> ()  [unwired: 1 in, 6 out]
            n341 = call "AOTFSettings.vi"() -> ("AOTF Setting (Output)"=w397:T14)  [unwired: 2 in]
            n342 = call "AnalogSettings.vi"() -> ("Analog Settings (output)"=w398:T15)  [unwired: 2 in]
            n343 = Unbundle By Name(w398) -> ("PCI 671x Device Number"=w396:u32)
            n344 = Unbundle By Name(w397) -> ("Laser 4 Output Channel"=w395:tag, "AOTF  4 Output Voltage"=w394:dbl)
            n345 = case shown="True" "Laser 4" {
              tunnel: w396 -> [w399 w404]
              tunnel: w395 -> [w400 w403]
              tunnel: w394 -> [_ w402]
              frame #0 {
                n346 = call-poly "AO Update Channel (scaled value).vi"("value"=sgl 0.0, "channel (0)"=w400, "device"=w399) -> ()
              }
              frame #1 {
                n347 = call-poly "AO Update Channel (scaled value).vi"("value"=w402, "channel (0)"=w403, "device"=w404) -> ()
              }
            }
          }
          event #16 {
            n348 = event-data() -> ()  [unwired: 1 in, 5 out]
            n349 = stacked-sequence {
              frame #0 {
                n350 = call "offset.vi"("set?"=TRUE, "offset"="offset (pixel)") -> ()  [unwired: 1 in, 1 out]
              }
              frame #1 {
                n351 = property on="Image Settings" class="Clust (strict)"() -> ("Value"=w407:T10)  [unwired: 2 in, 2 out]
                n352 = call "UpdateDestroyPositionJustOffset.vi"("Image Settings"=w407) -> ("error out"=w408:errorcluster)  [unwired: 1 in]
                n353 = call "HandleError.vi"("error in (no error)"=w408) -> ()
              }
            }
          }
          event #17 {
            n354 = event-data() -> ()  [unwired: 1 in, 5 out]
            n355 = call "PickImage.vi"() -> ("Image (output)"=w412:T7)  [unwired: 2 in]
            n356 = Unbundle By Name(w412) -> ("Rawdata"=w411:T6, "Mask"=w410:T6, "Display"=w409:T6)
            n357 = call "IMAQ Dispose"("Image"=w411) -> ()  [unwired: 5 in, 1 out]
            n358 = call "IMAQ Dispose"("Image"=w410) -> ()  [unwired: 5 in, 1 out]
            n359 = call "IMAQ Dispose"("Image"=w409) -> ()  [unwired: 5 in, 1 out]
          }
        }
      }
    }
  }
